vi "Set Targets.vi"(10 "Targets":refnum<vi>[](array[refnum]), 11 "Project Sync Tools in":refnum<class "Project Sync Tools.lvclass">) -> (3 "Project Sync Tools out":refnum<class "Project Sync Tools.lvclass">)   [LabVIEW 2019, in "Project Sync Tools.lvclass"]
uses:
  Project Sync Tools.lvclass
  Project Sync Tools.lvclass/Project Sync Tools.ctl
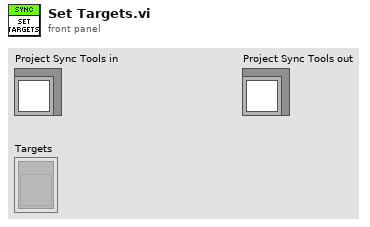
[diagram p1: front panel]
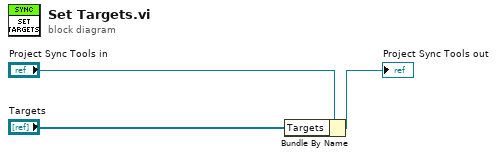
[diagram p0: block diagram]
diagram:
  n1 = Bundle By Name(cluster="Project Sync Tools in", "Targets"="Targets") -> (→"Project Sync Tools out":refnum<class "Project Sync Tools.lvclass">)
